vi "Magnet Rotation.vi"(8 "error in (no error)":errorcluster, 9 "Timeout (sec)":dbl=8.0, 10 "Hardware Parameters":T2={"Scan Calibration [G/V]"=0.0, "Modulation Calibration [G/V]"=0.0, "Modulation Phase [deg]"=0.0, "Modulation Frequency [Hz]"=0.0, "Attenuation [dB]"=0, "Input Channel Count"=0, "Time constant"=7, "Sensitivity"=17, "Frequency Output Voltage [V]"=0.0, "Phase Output Voltage [V]"=0.0, "Lock-in Offset Compensation"=FALSE, "RF [GHz]"=0.0, "Q Start"=0.0, "Q End"=0.0, "Balance"=0.0, "Phase Error"=0.0, "AFC Error"=0.0, "AFC"=FALSE, "Magnet Rotation"=FALSE, "Balance Scaling Factor"=1.0, "Phase Error Scaling Factor"=1.0, "AFC Error Scaling Factor"=1.0, "Frequency Counter ID"="", "Sweep Waveform"=enum."Sawtooth", "Q-Factor Scale"=0.0, " Q-Data Scale"=0.0, " Q-Data Offset"=0.0, "Magnet Rotation Slope"=0.0, "Magnet Rotation Offset"=0.0, "Phase Sweep Resolution"=0.0, "Hardware Version Number"="", "Spectrometer ID Number"=0, "Spectrometer Name"="", "Lock in Saturation"=0.0, "Balance Threshold"=0.0, "Phase Error Threshold"=0.0, "AFC Error Threshold"=0.0, "Linear Actuator Length"=0.0, "Lock-in OK?"=FALSE, "Ignore Lock-in Comm. Failure"=FALSE, "Gradient Addresses"=[], "Gradient Calibrations [G/A*mm]"=[], "Gradient Power Supplies"=[], "Lock-in Address"="", "Magnet Type"=enum."RRI", "Camera Names"=[], "Sweep Limit [Gauss]"=0.0, "Modulation Limit [Gauss]"=0.0, "Balance Threshold Exceeded?"=FALSE, "Phase Threshold Exceeded?"=FALSE, "AFC Threshold Exceeded?"=FALSE, "Consecutive Re-tune attempts"=0, "Reverse Sweep Slope [sec]"=0.0, "Reverse Sweep Offset [G]"=0.0, "AFC Field Correction [V/MHz]"=0.0, "Active Gradients (X Y Z)"=[], "SpO2 Calibration [SpO2/V]"=1.0, "Heart Rate Calibration [BPM/V]"=1.0, "Thermocouple Channel"=""} {"Sensitivity" items=["", "2 nV", "5 nV", "10 nV", "20 nV", "50 nV", "100 nV", "200 nV", "500 nV", "1 uV", "2 uV", "5 uV", "10 uV", "20 uV", "50 uV", "100 uV", "200 uV", "500 uV", "1 mV", "2 mV", "5 mV", "10 mV", "20 mV", "50 mV", "100 mV", "200 mV", "500 mV", "1 V"]; "Time constant" items=["10 us", "20 us", "40 us", "80 us", "160 us", "320 us", "640 us", "5 ms", "10 ms", "20 ms", "50 ms", "100 ms", "200 ms", "500 ms", "1 s", "2 s", "5 s", "10 s", "20 s", "50 s", "100 s", "200 s", "500 s", "1 ks", "2 ks", "5 ks", "10 ks", "20 ks", "50 ks", "100 ks"]}, 11 "Acquisition Parameters":T1={"Magnet Angle [deg]"=0.0, "Magnet Angles [deg]"=[], "DeltaVpp [v]"=0.0, "SEM [v]"=0.0, "DeltaVpp Thresh [v]"=0.0, "SEM Thresh [v]"=0.0, "Adaptive Processing"=FALSE, "Acquire Q"=FALSE, "Acquire Photos"=FALSE, "Adaptive Tuning"=FALSE, "Automated Matching"=FALSE, "X-Gradient [G/mm]"=0.0, "Y-Gradient [G/mm]"=0.0, "Z-Gradient [G/mm]"=0.0, "Central Field [G]"=0.0, "Scan Width [G]"=0.0, "Mod. Amp. [G]"=0.0, "Scan Time [s]"=0.0, "Pre-Scan Delay [ms]"=0, "Measurement Timeout [s]"=0.0, "Electromagnet Main Field [G]"=0.0, "Locked Central Field [G]"=0.0, "Scans Excluded"=0, "Scans Completed"=0, "No. Scans/Set"=0, "No. Scans for SNR"=0, "Field Locked Frequency [GHz]"=0.0, "Auto Set-based Field Center"=FALSE, "Prompt for oxy acquisition updates"=FALSE, "Oxy QA Scan?"=FALSE, "Exclude Bad Data"=FALSE, "Optimizing RF Power"=FALSE, "Gradients on/off"=FALSE, "Running Script"=TRUE, "Opto-Coupler Current [A]"=0.0, "Continuous Sweeping"=FALSE, "Sweep Rise Time [sec]"=0, "Reverse Sweep Central Field [G]"=0.0, "Forward Sweep Central Field [G]"=0.0, "Sweep Calibrated"=FALSE, "Modulation Calibrated"=FALSE, "First CheckCal Scan?"=FALSE, "AFC Field Correction"=FALSE, "OxyQAInit Scan Width [G]"=0.0, "OxyQAInit Mod. Amp. [G]"=0.0, "Scans Completed/Session"=0, "Acquire SpO2"=FALSE, "Acquire Temperature"=FALSE, "Over Mod"=FALSE} {"OxyQAInit Mod. Amp. [G]" min=0.0; "OxyQAInit Scan Width [G]" min=0.0; "Mod. Amp. [G]" min=0.0; "Scan Width [G]" min=0.0; "Central Field [G]" min=0.0; "Measurement Timeout [s]" min=0.0; "Scan Time [s]" min=0.0; "Z-Gradient [G/mm]" min=0.0; "SEM Thresh [v]" min=0.0; "SEM [v]" min=0.0; "DeltaVpp [v]" min=0.0}) -> (0 "error out":errorcluster, 3 "Achieved Desired Position":bool=TRUE)   [LabVIEW 2016]
uses:
  Types/Hardware Parameters.ctl
  Types/Acquisition Parameters.ctl
panel:
  in  "Actuator Length [mm]":dbl format="%.2f"
  out "Actual Angle (deg)":dbl=-0.04071752981920655
  in  "Desired Angle (deg)":dbl min=-9.0 max=9.0
  in  "Use Rotation Calibration?":bool=TRUE
  in  "Rotation Platform Intercept":dbl=48.798
  in  "Rotation Platform Slope":dbl=5.2901
  in  "Stop":bool
  out "Actual Position (mm)":dbl=48.58260019550342
  in  "Desired Position (mm)":dbl min=0.0 max=100.0 step=0.01
  # "Gradients"
  # "Field"
  # "Scans and Sets"
  # "Timing"
  # "Adaptive Dosimetric \nData Processing"
  # "Bridge I/O"
  # "Magnet Rotation"
  # "Field Calibration"
  # "Lock In Amplifier"
  # "Spectrometer Information"
  # "DAQ Settings"
  # "Gradient Coils and Field"
  # "X"
  # "Y"
  # "Z"
  # "Q-Measurements"
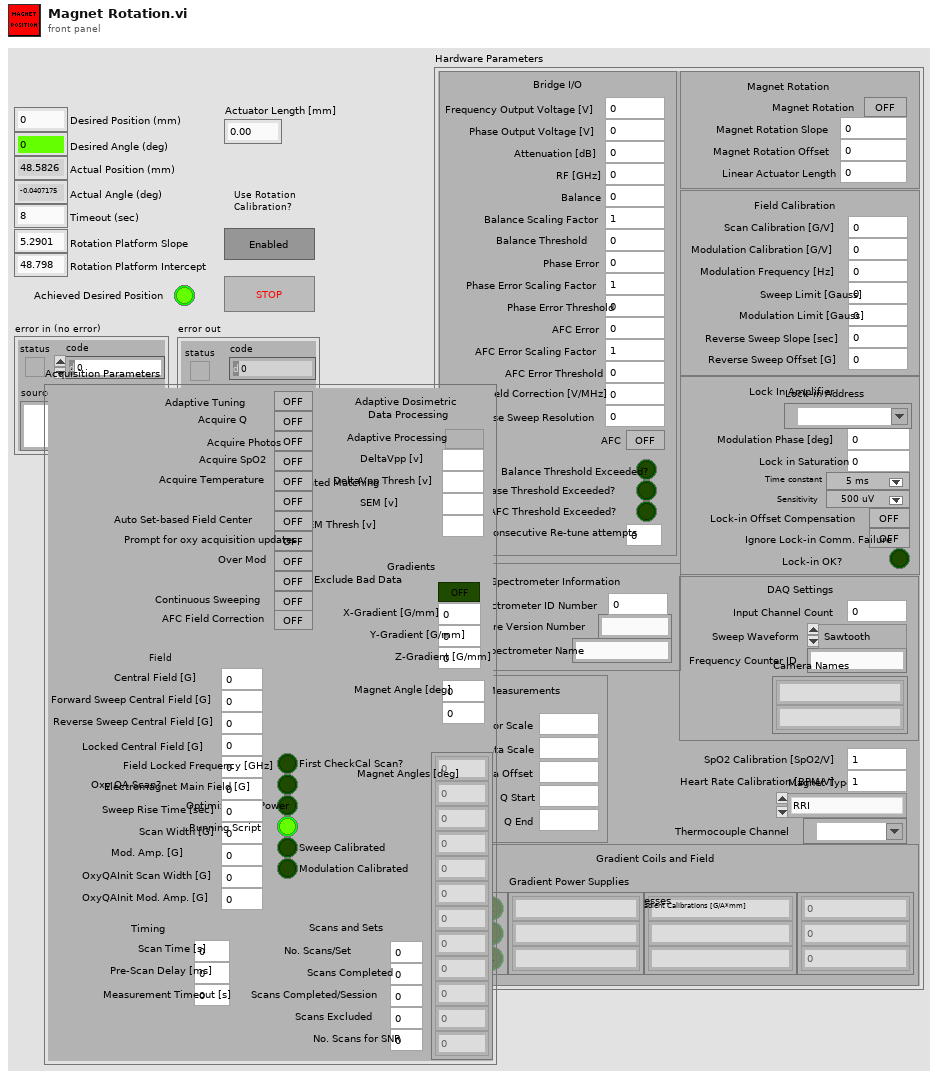
[diagram p1: front panel]
types:
  T1 = typedef "Acquisition Parameters.ctl" = cluster{"Magnet Angle [deg]":dbl, "Magnet Angles [deg]":dbl[], "DeltaVpp [v]":dbl, "SEM [v]":dbl, "DeltaVpp Thresh [v]":dbl, "SEM Thresh [v]":dbl, "Adaptive Processing":bool, "Acquire Q":bool, "Acquire Photos":bool, "Adaptive Tuning":bool, "Automated Matching":bool, "X-Gradient [G/mm]":dbl, "Y-Gradient [G/mm]":dbl, "Z-Gradient [G/mm]":dbl, "Central Field [G]":dbl, "Scan Width [G]":dbl, "Mod. Amp. [G]":dbl, "Scan Time [s]":dbl, "Pre-Scan Delay [ms]":u32, "Measurement Timeout [s]":dbl, "Electromagnet Main Field [G]":dbl, "Locked Central Field [G]":dbl, "Scans Excluded":u32, "Scans Completed":u32, "No. Scans/Set":u32, "No. Scans for SNR":u32, "Field Locked Frequency [GHz]":dbl, "Auto Set-based Field Center":bool, "Prompt for oxy acquisition updates":bool, "Oxy QA Scan?":bool, "Exclude Bad Data":bool, "Optimizing RF Power":bool, "Gradients on/off":bool, "Running Script":bool, "Opto-Coupler Current [A]":dbl, "Continuous Sweeping":bool, "Sweep Rise Time [sec]":u32, "Reverse Sweep Central Field [G]":dbl, "Forward Sweep Central Field [G]":dbl, "Sweep Calibrated":bool, "Modulation Calibrated":bool, "First CheckCal Scan?":bool, "AFC Field Correction":bool, "OxyQAInit Scan Width [G]":dbl, "OxyQAInit Mod. Amp. [G]":dbl, "Scans Completed/Session":u32, "Acquire SpO2":bool, "Acquire Temperature":bool, "Over Mod":bool}
  T2 = typedef "Hardware Parameters.ctl" = cluster{"Scan Calibration [G/V]":dbl, "Modulation Calibration [G/V]":dbl, "Modulation Phase [deg]":dbl, "Modulation Frequency [Hz]":dbl, "Attenuation [dB]":u16, "Input Channel Count":i32, "Time constant":u16, "Sensitivity":u16, "Frequency Output Voltage [V]":dbl, "Phase Output Voltage [V]":dbl, "Lock-in Offset Compensation":bool, "RF [GHz]":dbl, "Q Start":dbl, "Q End":dbl, "Balance":dbl, "Phase Error":dbl, "AFC Error":dbl, "AFC":bool, "Magnet Rotation":bool, "Balance Scaling Factor":dbl, "Phase Error Scaling Factor":dbl, "AFC Error Scaling Factor":dbl, "Frequency Counter ID":string, "Sweep Waveform":enum16{"Sine Wave", "Square Wave", "Sawtooth", "Triangle Wave"}, "Q-Factor Scale":dbl, " Q-Data Scale":dbl, " Q-Data Offset":dbl, "Magnet Rotation Slope":dbl, "Magnet Rotation Offset":dbl, "Phase Sweep Resolution":dbl, "Hardware Version Number":string, "Spectrometer ID Number":i32, "Spectrometer Name":string, "Lock in Saturation":dbl, "Balance Threshold":dbl, "Phase Error Threshold":dbl, "AFC Error Threshold":dbl, "Linear Actuator Length":dbl, "Lock-in OK?":bool, "Ignore Lock-in Comm. Failure":bool, "Gradient Addresses":string[], "Gradient Calibrations [G/A*mm]":dbl[], "Gradient Power Supplies":string[], "Lock-in Address":refnum<visa-resource-name>, "Magnet Type":enum16{"RRI", "BARDA", "Whole Body Permanent", "RRI Electromagnet"}, "Camera Names":string[], "Sweep Limit [Gauss]":dbl, "Modulation Limit [Gauss]":dbl, "Balance Threshold Exceeded?":bool, "Phase Threshold Exceeded?":bool, "AFC Threshold Exceeded?":bool, "Consecutive Re-tune attempts":i32, "Reverse Sweep Slope [sec]":dbl, "Reverse Sweep Offset [G]":dbl, "AFC Field Correction [V/MHz]":dbl, "Active Gradients (X Y Z)":bool[], "SpO2 Calibration [SpO2/V]":dbl, "Heart Rate Calibration [BPM/V]":dbl, "Thermocouple Channel":tag}
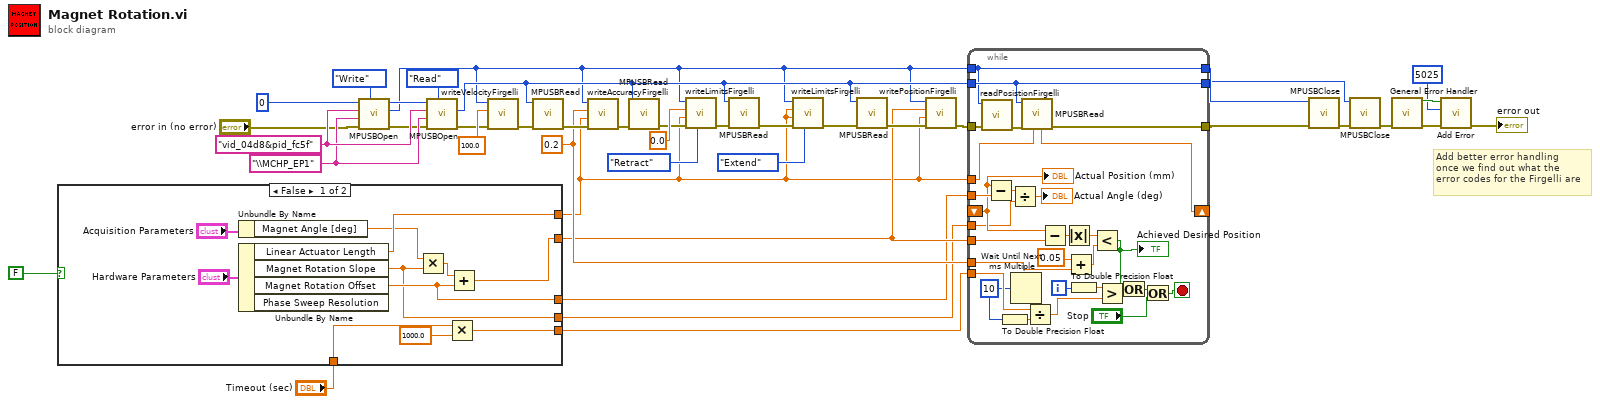
[diagram p0: block diagram]
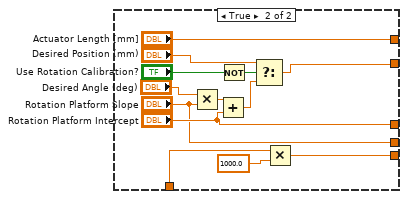
[diagram p2: hidden frame]
diagram:
  w12 = 0.2 ("Accuracy")
  w39 = "\\MCHP_EP1" ("pEP")
  w40 = "vid_04d8&pid_fc5f"
  # "Add better error handling\nonce we find out what the \nerror codes for the Firgelli are"
  n1 = case shown="False" FALSE {
    tunnel: [w45 w64] -> w11
    tunnel: [w49 w58] -> w10
    tunnel: [w48 "Rotation Platform Intercept"] -> w9
    tunnel: [w47 "Rotation Platform Slope"] -> w8
    tunnel: [w51 "Actuator Length [mm]"] -> w7
    tunnel: "Timeout (sec)" -> [w42 w53]
    frame False {
      n2 = Unbundle By Name("Acquisition Parameters") -> ("Magnet Angle [deg]"=w43:dbl)
      n3 = Unbundle By Name("Hardware Parameters") -> ("Linear Actuator Length"=w51:dbl, "Magnet Rotation Slope"=w47:dbl, "Magnet Rotation Offset"=w48:dbl)  [unwired: 1 out]
      n4 = Multiply(x=w43, y=w47) -> (x*y=w50:dbl)
      n5 = Multiply(x=w42, y=1000.0) -> (x*y=w45:dbl)
      n6 = Add(x=w50, y=w48) -> (x+y=w49:dbl)
    }
    frame True {
      n7 = Multiply(x="Desired Angle (deg)", y="Rotation Platform Slope") -> (x*y=w63:dbl)
      n8 = Add(x=w63, y="Rotation Platform Intercept") -> (x+y=w62:dbl)
      n9 = Not(x="Use Rotation Calibration?") -> (.not. x?=w61:bool)
      n10 = Select(t="Desired Position (mm)", s=w61, f=w62) -> (s? t:f=w58:dbl)
      n11 = Multiply(x=w53, y=1000.0) -> (x*y=w64:dbl)
    }
  }
  n12 = call "MPUSBOpen.vi"("dwDir"=enum16{"Write", "Read"}."Write", "error in (no error)"="error in (no error)", "pEP"=w39, "pVID_PID"=w40, "instance"=u32 0 ("Instance")) -> ("error out"=w36:errorcluster, "HANDLE"=w15:u32, "instanceOut"=w34:u32)  [unwired: 4 in]
  n13 = call "MPUSBOpen.vi"("dwDir"=enum16{"Write", "Read"}."Read", "error in (no error)"=w36, "pEP"=w39, "pVID_PID"=w40, "instance"=w34) -> ("error out"=w27:errorcluster, "HANDLE"=w16:u32)  [unwired: 3 in, 2 out]
  n14 = call "writeVelocityFirgelli.vi"("error in (no error)"=w27, "Velocity"=100.0, "handleIn"=w15) -> ("error out"=w31:errorcluster)  [unwired: 8 out]
  n15 = call "MPUSBRead.vi"("error in (no error)"=w31, "handleIn"=w16) -> ("error out"=w28:errorcluster)  [unwired: 4 in, 5 out]
  n16 = call "writeAccuracyFirgelli.vi"("error in (no error)"=w28, "maxLength"=w7, "accuracy"=w12, "handleIn"=w15) -> ("error out"=w29:errorcluster)  [unwired: 7 out]
  n17 = call "MPUSBRead.vi"("error in (no error)"=w29, "handleIn"=w16) -> ("error out"=w20:errorcluster)  [unwired: 4 in, 5 out]
  n18 = call "writeLimitsFirgelli.vi"("select"=enum16{"Retract", "Extend"}."Retract", "error in (no error)"=w20, "maxLength"=w7, "limit"=0.0 ("minLength"), "handleIn"=w15) -> ("error out"=w23:errorcluster)  [unwired: 6 out]
  n19 = call "MPUSBRead.vi"("error in (no error)"=w23, "handleIn"=w16) -> ("error out"=w22:errorcluster)  [unwired: 4 in, 5 out]
  n20 = call "writeLimitsFirgelli.vi"("select"=enum16{"Retract", "Extend"}."Extend", "error in (no error)"=w22, "maxLength"=w7, "limit"=w7, "handleIn"=w15) -> ("error out"=w26:errorcluster)  [unwired: 6 out]
  n21 = call "MPUSBRead.vi"("error in (no error)"=w26, "handleIn"=w16) -> ("error out"=w18:errorcluster)  [unwired: 4 in, 5 out]
  n22 = call "writePositionFirgelli.vi"("error in (no error)"=w18, "lengthMax"=w7, "Position (mm)"=w10, "handleIn"=w15) -> ("error out"=w19:errorcluster)  [unwired: 7 out]
  n23 = while {
    tunnel: w19 -> [w91]
    tunnel: [w94] -> w17
    tunnel: w16 -> [w92]
    tunnel: w7 -> [w93]
    tunnel: w15 -> [w89]
    tunnel: [w89] -> w14
    tunnel: [w92] -> w13
    shift-right: [w88] -> _
    shift-left: _ -> [w71]
    tunnel: w10 -> [w87]
    tunnel: w12 -> [w84]
    tunnel: w11 -> [w76]
    tunnel: w9 -> [w72]
    tunnel: w8 -> [w69]
    i -> [w67]
    stop <- w78 stop-if-true
    w74 = u32 10 ("milliseconds to wait")
    n24 = call "readPosistionFirgelli.vi"("error in (no error)"=w91, "handleIn"=w89) -> ("error out"=w90:errorcluster)  [unwired: 9 out]
    n25 = Subtract(x=w71, y=w72) -> (x-y=w70:dbl)
    n26 = To Double Precision Float(number=w74) -> (double precision float=w75:dbl)
    n27 = Divide(x=w70, y=w69) -> (x/y=→"Actual Angle (deg)":dbl)
    n28 = Wait Until Next ms Multiple(millisecond multiple=w74) -> ()  [unwired: 1 out]
    n29 = call "MPUSBRead.vi"("maxLength"=w93, "error in (no error)"=w90, "handleIn"=w92) -> ("error out"=w94:errorcluster, "setValue"=w88:dbl)  [unwired: 3 in, 4 out]
    n30 = Divide(x=w76, y=w75) -> (x/y=w77:dbl)
    n31 = Subtract(x=w71, y=w87) -> (x-y=w86:dbl)
    n32 = Absolute Value(x=w86) -> (abs(x)=w85:dbl)
    n33 = Add(x=0.05, y=w84) -> (x+y=w82:dbl)
    n34 = To Double Precision Float(number=w67) -> (double precision float=w66:dbl)
    n35 = Less?(x=w85, y=w82) -> (x < y?=w73:bool)
    "Achieved Desired Position" <- w73
    n36 = Greater?(x=w66, y=w77) -> (0:w81:bool)
    n37 = Or(x=w73, y=w81) -> (x .or. y?=w80:bool)
    n38 = Or(x=w80, y="Stop") -> (x .or. y?=w78:bool)
    "Actual Position (mm)" <- w71
  }
  n39 = call "MPUSBClose.vi"("error in (no error)"=w17, "handle"=w14) -> ("error out"=w35:errorcluster)  [unwired: 1 in, 8 out]
  n40 = call "MPUSBClose.vi"("error in (no error)"=w35, "handle"=w13) -> ("error out"=w41:errorcluster)  [unwired: 1 in, 8 out]
  n41 = call <vilib>:"General Error Handler.vi"("error in (no error)"=w41) -> ("error?"=w4:bool, "error out"=w3:errorcluster)  [unwired: 2 in, 11 out]
  n42 = call "Add Error.vi"("error in (no error)"=w3, "error code (0)"=5025, "error?"=w4) -> ("error out"=→"error out":errorcluster)  [unwired: 8 in]
